vi "Plot a Circle.vi"() -> ()   [LabVIEW 2018]
panel:
  out "XY Graph":cluster{dbl[], dbl[]}(graph)
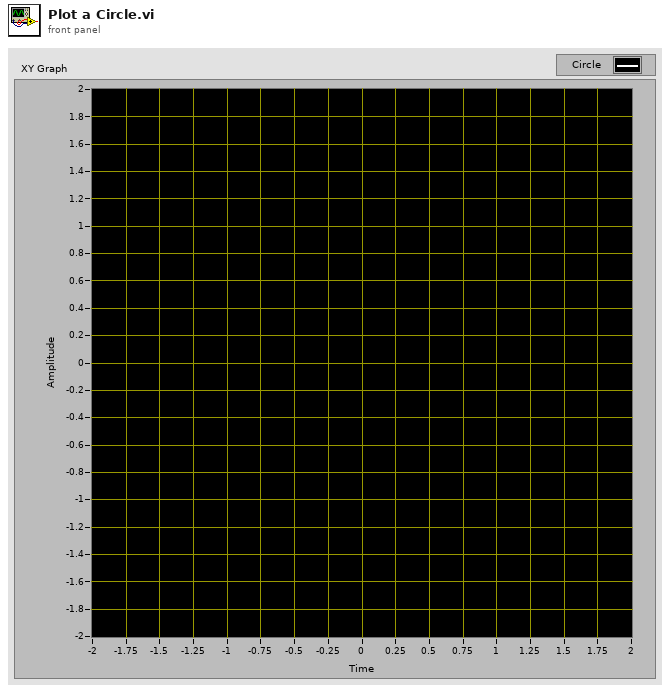
[diagram p1: front panel]
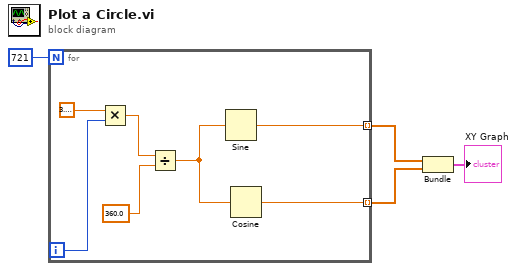
[diagram p0: block diagram]
diagram:
  n1 = for {
    N: 721 -> [_]
    tunnel: [w9] -> w3 mode=indexing
    tunnel: [w8] -> w2 mode=indexing
    i -> [w10]
    n2 = Multiply(x=3.141592653589793, y=w10) -> (x*y=w7:dbl)
    n3 = Divide(x=w7, y=360.0) -> (x/y=w6:dbl)
    n4 = Sine(x=w6) -> (sin(x)=w9:dbl)
    n5 = Cosine(x=w6) -> (cos(x)=w8:dbl)
  }
  n6 = Bundle(w3, w2) -> (→"XY Graph":cluster{dbl[], dbl[]})  [unwired: 1 in]
